vi "swiatla drogowe.vi"() -> ()   [LabVIEW 2025]
uses:
  Semafor1.ctl
  zmienna stanu.ctl
panel:
  in  "OK Button":bool
  out "error out":errorcluster
  in  "number":dbl
  in  "file path (use dialog)":path=path "C:/Users/33sbx/Documents/LABVIEW/światła drogowe/raport.txt"
  out "concatenated string":string
  in  "Zapisz":bool
  out "S4":T1
  out "Obecna sekwencja":T2
  out "S3":T1
  out "S2":T1
  out "S1":T1
  out "Waveform Chart":dbl(graph)
  in  "Reset":bool
  out "Parametr J":dbl
  in  "STOP":bool
  out "OPC22":bool
  out "OPC21":bool
  out "OPZ21":bool
  out "OPZ22":bool
  in  "OPA22":bool
  in  "OPA21":bool
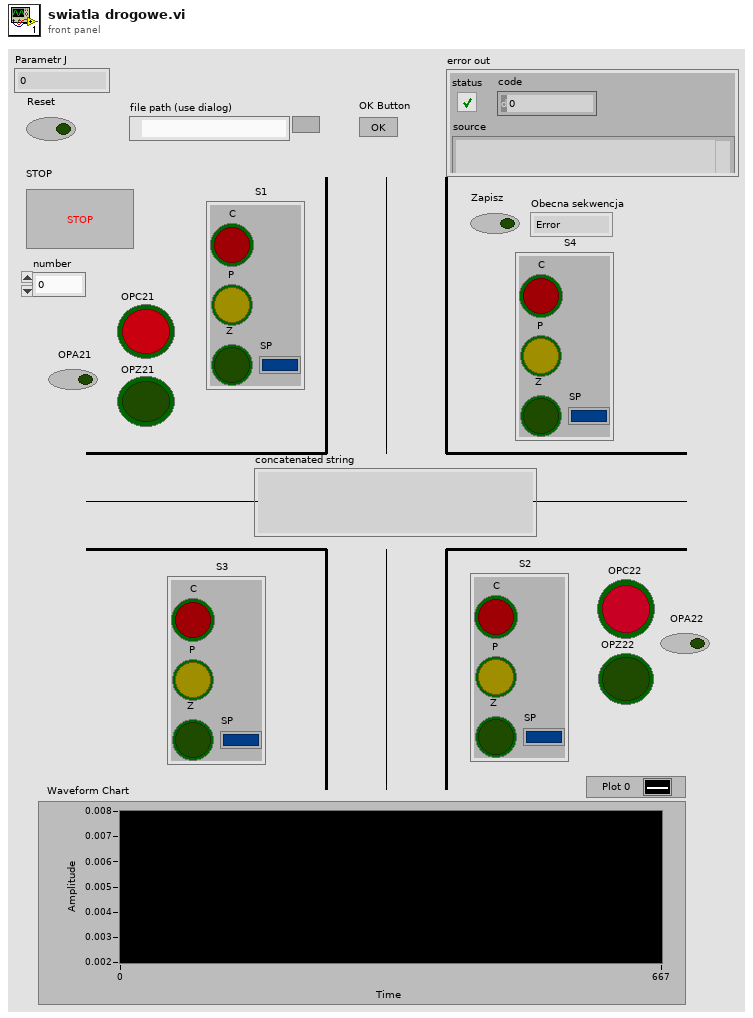
[diagram p1: front panel]
types:
  T1 = typedef "Semafor1.ctl" = cluster{"C":bool, "P":bool, "Z":bool, "SP":bool}
  T2 = typedef "zmienna stanu.ctl" = enum16{"Error", "KGczerwony", "KGpomarañczowy", "KGzielony", "KGpom-czer", "KPpom-czer", "KPzielony", "KPpomarañczowy", "KGczerwony2", "KPpom-czer2", "AwariaON", "AwariaOFF", ""}
  T3 = enum16{"open", "replace", "create", "open or create", "replace or create", "replace or create with confirmation"}
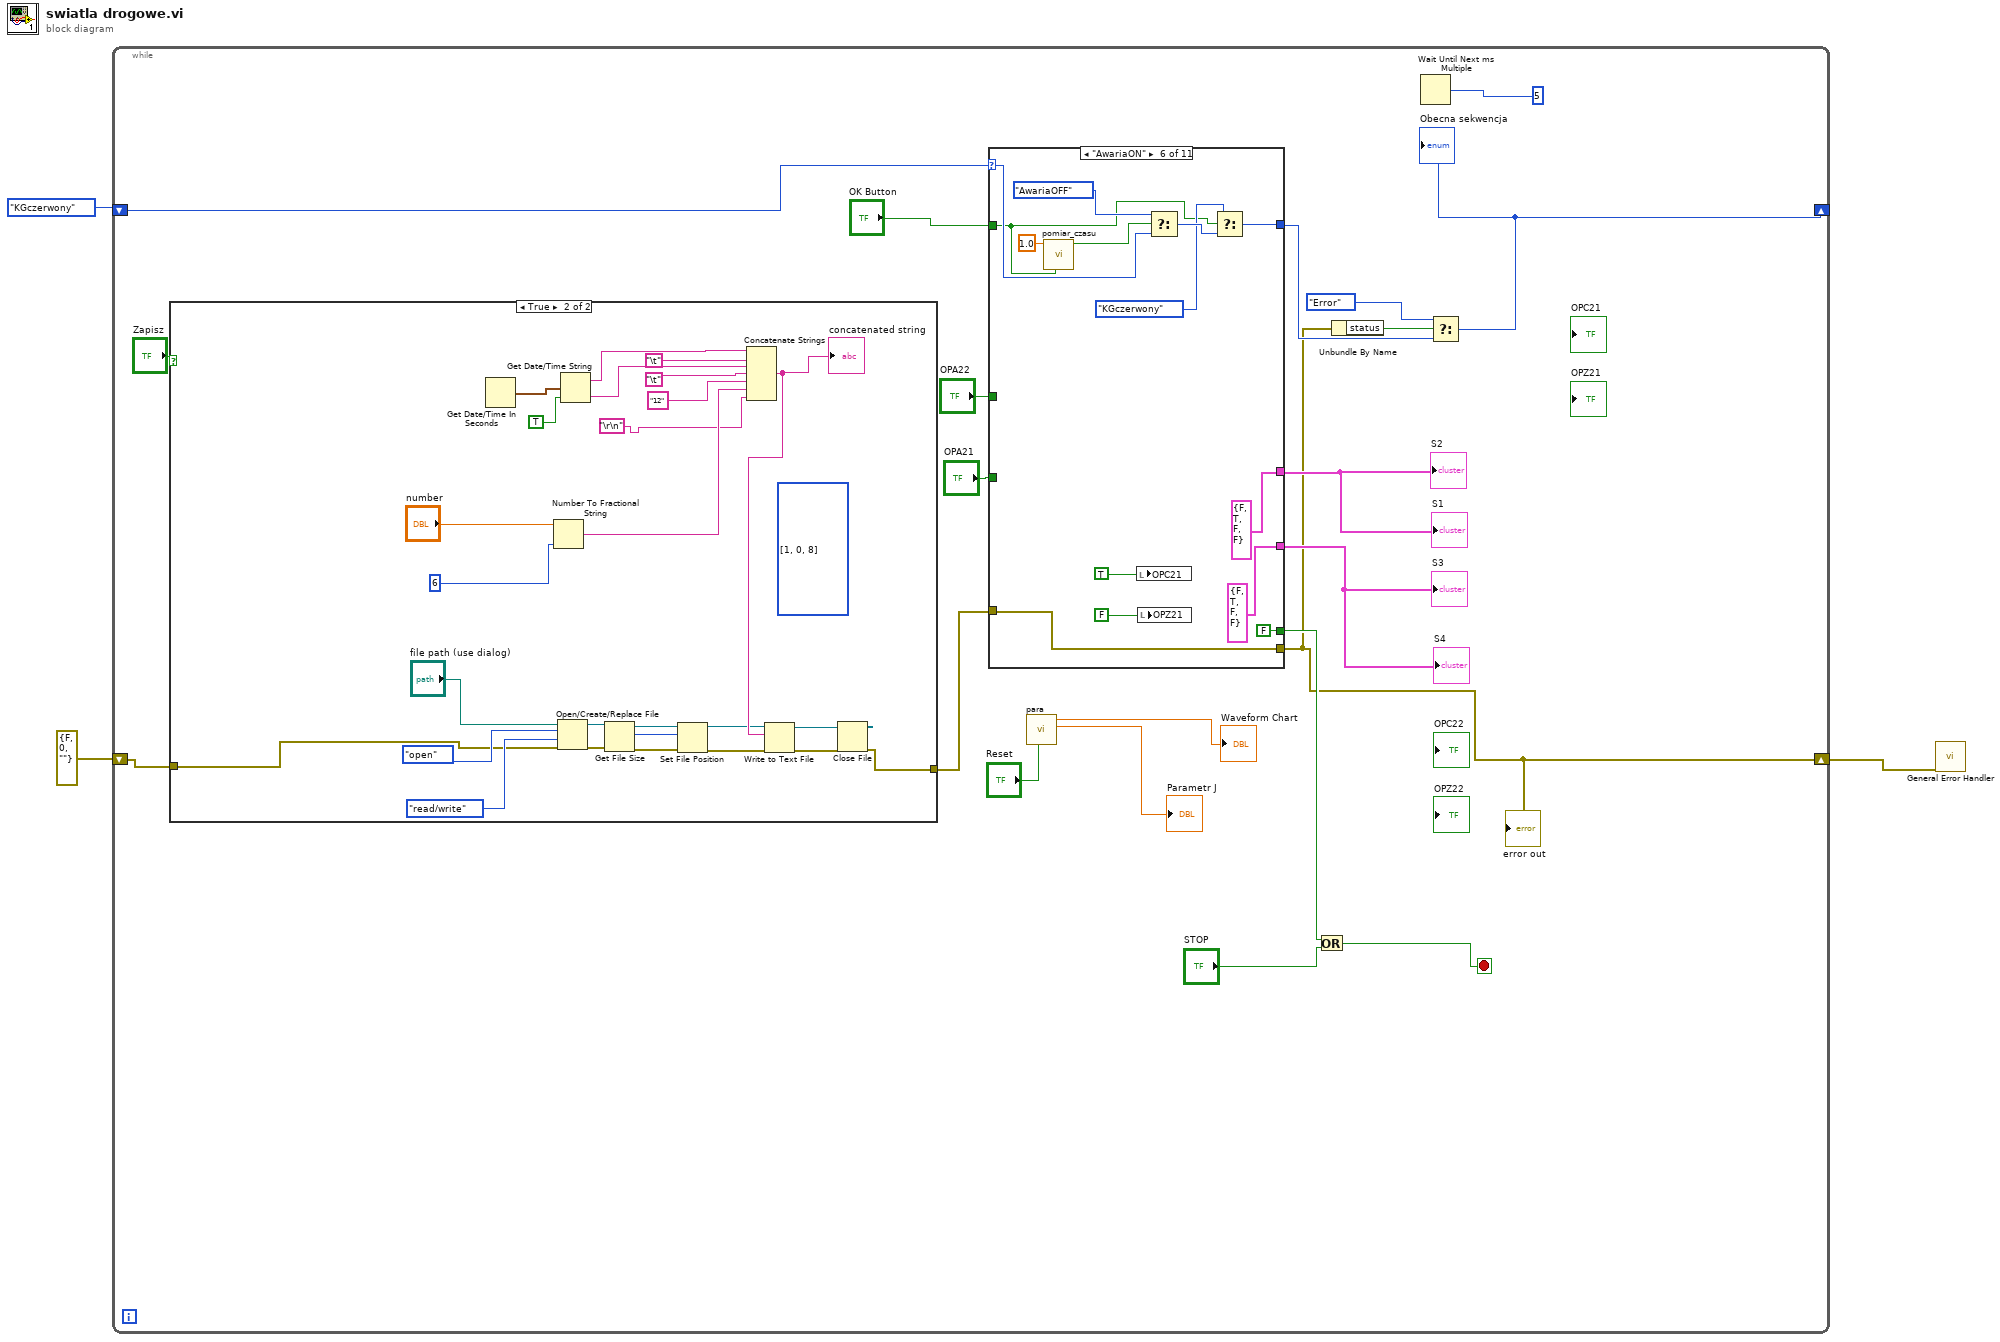
[diagram p0: block diagram]
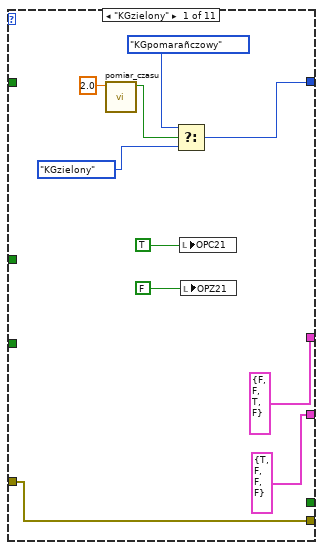
[diagram p3: hidden frame]
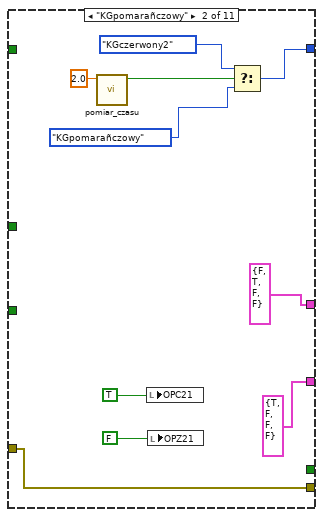
[diagram p4: hidden frame]
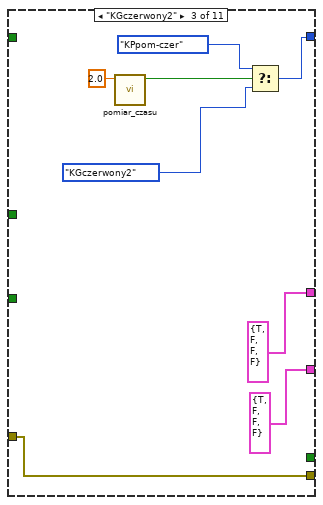
[diagram p5: hidden frame]
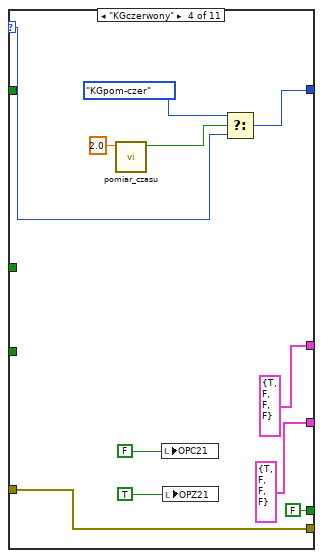
[diagram p6: hidden frame]
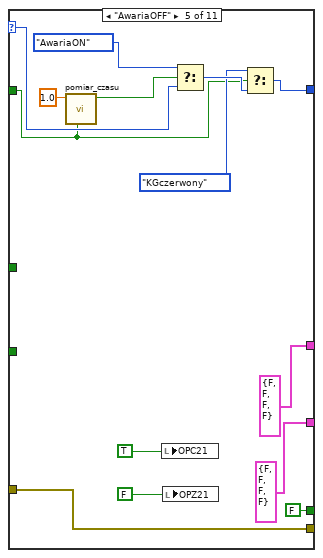
[diagram p7: hidden frame]
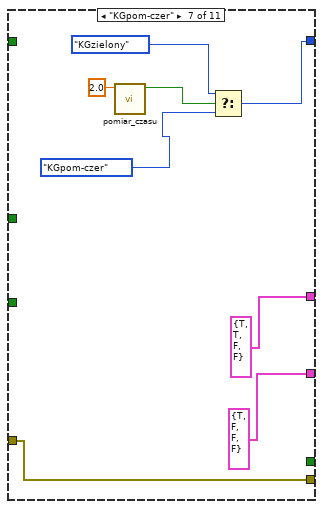
[diagram p8: hidden frame]
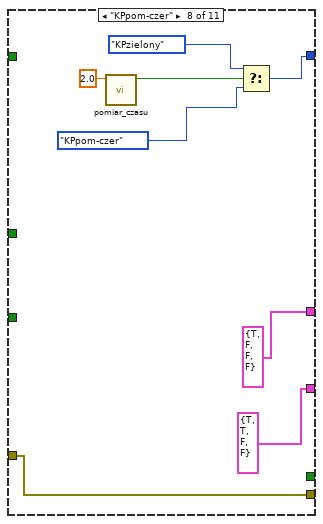
[diagram p9: hidden frame]
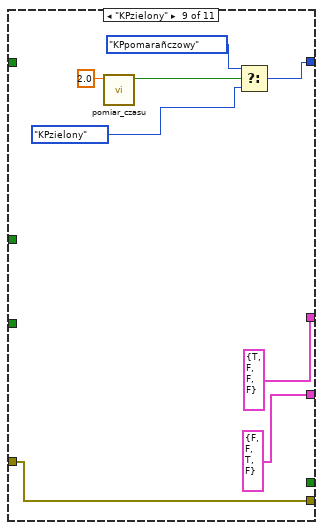
[diagram p10: hidden frame]
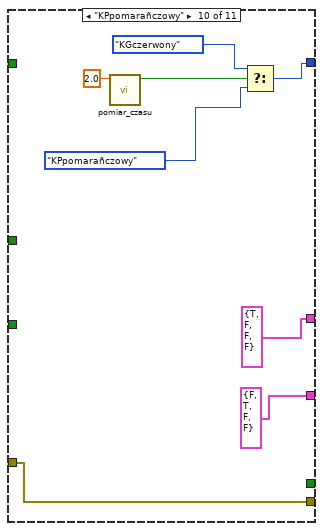
[diagram p11: hidden frame]
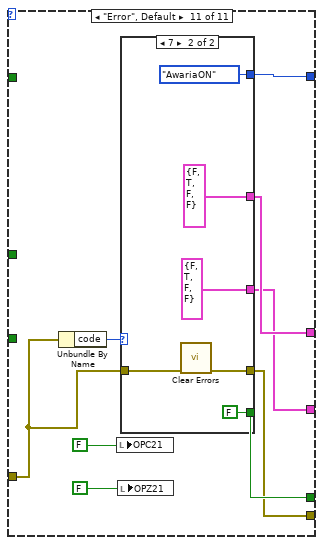
[diagram p12: hidden frame]
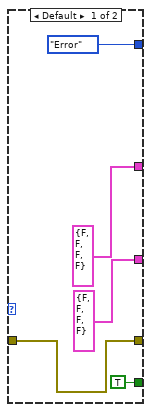
[diagram p13: hidden frame]
diagram:
  n1 = while {
    shift-right: [w10] -> _
    shift-left: zmienna_stanu."KGczerwony" -> [w23]
    shift-right: [w5] -> w1
    shift-left: errorcluster {"status"=FALSE, "code"=0, "source"=""} ("error constant") -> [w13]
    stop <- w7 stop-if-true
    n2 = case shown="True" "Zapisz" {
      tunnel: [w25 w26] -> w14
      tunnel: w13 -> [w25 w31]
      frame False {
      }
      frame True {
        (unwired) u8[] [1, 0, 8]
        n3 = Get Date/Time In Seconds() -> (seconds since 1Jan1904=w51:timestamp)
        n4 = Number To Fractional String(number="number", precision (6)=i16 6) -> (F-format string=w33:string)  [unwired: 2 in]
        n5 = Open/Create/Replace File(file path (use dialog)="file path (use dialog)", error in=w31, operation (0:open)=T3."open", access (0:read/write)=enum16{"read/write", "read-only", "write-only"}."read/write") -> (refnum out=w41:refnum<file>, error out=w30:errorcluster)  [unwired: 2 in, 1 out]
        n6 = Get Date/Time String(seconds (now)=w51, want seconds? (F)=TRUE) -> (date string=w45:string, time string=w48:string)  [unwired: 1 in]
        n7 = Get File Size(file=w41, error in=w30) -> (refnum out=w39:refnum<file>, size (in bytes)=w38:i64, 0:w29:errorcluster)
        n8 = Set File Position(offset (in bytes) (0)=w38, refnum=w39, error in=w29) -> (refnum out=w37:refnum<file>, error out=w28:errorcluster)  [unwired: 1 in]
        n9 = Concatenate Strings(w45, "\t", w48, "\t", "12" ("string"), w33, "\r\n") -> (w42:string)
        "concatenated string" <- w42
        n10 = Write to Text File(file (use dialog)=w37, text=w42, error in=w28) -> (refnum out=w40:refnum<file>, error out=w27:errorcluster)  [unwired: 1 in, 1 out]
        n11 = Close File(refnum=w40, error in=w27) -> (error out=w26:errorcluster)  [unwired: 1 out]
      }
    }
    n12 = case shown="\"AwariaON\"" w23 {
      selector: w23 -> [_ _ _ w84 w99 w113 _ _ _ _ _]
      tunnel: [w59 w68 w76 w85 w94 w106 w122 w129 w137 w147 w151] -> w11
      tunnel: "OPA21" -> [_ _ _ _ _ _ _ _ _ _ _]
      tunnel: [T1 {"C"=FALSE, "P"=FALSE, "Z"=TRUE, "SP"=FALSE} ("S1") T1 {"C"=FALSE, "P"=TRUE, "Z"=FALSE, "SP"=FALSE} ("S1") T1 {"C"=TRUE, "P"=FALSE, "Z"=FALSE, "SP"=FALSE} ("S1") T1 {"C"=TRUE, "P"=FALSE, "Z"=FALSE, "SP"=FALSE} ("S1") T1 {"C"=FALSE, "P"=FALSE, "Z"=FALSE, "SP"=FALSE} ("S1") T1 {"C"=FALSE, "P"=TRUE, "Z"=FALSE, "SP"=FALSE} ("S1") T1 {"C"=TRUE, "P"=TRUE, "Z"=FALSE, "SP"=FALSE} ("S1") T1 {"C"=TRUE, "P"=FALSE, "Z"=FALSE, "SP"=FALSE} ("S1") T1 {"C"=TRUE, "P"=FALSE, "Z"=FALSE, "SP"=FALSE} ("S1") T1 {"C"=TRUE, "P"=FALSE, "Z"=FALSE, "SP"=FALSE} ("S1") w157] -> w18
      tunnel: [T1 {"C"=TRUE, "P"=FALSE, "Z"=FALSE, "SP"=FALSE} ("S4") T1 {"C"=TRUE, "P"=FALSE, "Z"=FALSE, "SP"=FALSE} ("S4") T1 {"C"=TRUE, "P"=FALSE, "Z"=FALSE, "SP"=FALSE} ("S4") T1 {"C"=TRUE, "P"=FALSE, "Z"=FALSE, "SP"=FALSE} ("S4") T1 {"C"=FALSE, "P"=FALSE, "Z"=FALSE, "SP"=FALSE} ("S4") T1 {"C"=FALSE, "P"=TRUE, "Z"=FALSE, "SP"=FALSE} ("S4") T1 {"C"=TRUE, "P"=FALSE, "Z"=FALSE, "SP"=FALSE} ("S4") T1 {"C"=TRUE, "P"=TRUE, "Z"=FALSE, "SP"=FALSE} ("S4") T1 {"C"=FALSE, "P"=FALSE, "Z"=TRUE, "SP"=FALSE} ("S4") T1 {"C"=FALSE, "P"=TRUE, "Z"=FALSE, "SP"=FALSE} ("S4") w156] -> w17
      tunnel: "OPA22" -> [_ _ _ _ _ _ _ _ _ _ _]
      tunnel: [w52 w62 w72 w81 w96 w110 w119 w127 w135 w143 w152] -> w5
      tunnel: w14 -> [w52 w62 w72 w81 w96 w110 w119 w127 w135 w143 w153]
      tunnel: [_ _ _ FALSE ("x") FALSE ("x") FALSE ("x") _ _ _ _ w155] -> w8
      tunnel: "OK Button" -> [_ _ _ _ w91 w105 _ _ _ _ _]
      frame "KGzielony" {
        n13 = call "pomiar_czasu.vi"("czas do odmierzenia"=2.0) -> ("gotowe"=w55:bool)  [unwired: 9 in, 1 out]
        n14 = Select(t=zmienna_stanu."KGpomarañczowy", s=w55, f=zmienna_stanu."KGzielony") -> (s? t:f=w59:T2)
        n15 = local write "OPC21"(TRUE) -> ()
        n16 = local write "OPZ21"(FALSE) -> ()
      }
      frame "KGpomarañczowy" {
        n17 = call "pomiar_czasu.vi"("czas do odmierzenia"=2.0) -> ("gotowe"=w66:bool)  [unwired: 9 in, 1 out]
        n18 = local write "OPC21"(TRUE) -> ()
        n19 = local write "OPZ21"(FALSE) -> ()
        n20 = Select(t=zmienna_stanu."KGczerwony2", s=w66, f=zmienna_stanu."KGpomarañczowy") -> (s? t:f=w68:T2)
      }
      frame "KGczerwony2" {
        n21 = call "pomiar_czasu.vi"("czas do odmierzenia"=2.0) -> ("gotowe"=w78:bool)  [unwired: 9 in, 1 out]
        n22 = Select(t=zmienna_stanu."KPpom-czer", s=w78, f=zmienna_stanu."KGczerwony2") -> (s? t:f=w76:T2)
      }
      frame "KGczerwony" {
        n23 = call "pomiar_czasu.vi"("czas do odmierzenia"=2.0) -> ("gotowe"=w82:bool)  [unwired: 9 in, 1 out]
        n24 = local write "OPC21"(FALSE) -> ()
        n25 = local write "OPZ21"(TRUE) -> ()
        n26 = Select(t=zmienna_stanu."KGpom-czer", s=w82, f=w84) -> (s? t:f=w85:T2)
      }
      frame "AwariaOFF" {
        n27 = call "pomiar_czasu.vi"("Reset"=w91, "czas do odmierzenia"=1.0) -> ("gotowe"=w97:bool)  [unwired: 8 in, 1 out]
        n28 = local write "OPC21"(TRUE) -> ()
        n29 = local write "OPZ21"(FALSE) -> ()
        n30 = Select(t=zmienna_stanu."AwariaON", s=w97, f=w99) -> (s? t:f=w93:T2)
        n31 = Select(t=zmienna_stanu."KGczerwony", s=w91, f=w93) -> (s? t:f=w94:T2)
      }
      frame "AwariaON" {
        n32 = call "pomiar_czasu.vi"("Reset"=w105, "czas do odmierzenia"=1.0) -> ("gotowe"=w111:bool)  [unwired: 8 in, 1 out]
        n33 = local write "OPC21"(TRUE) -> ()
        n34 = local write "OPZ21"(FALSE) -> ()
        n35 = Select(t=zmienna_stanu."AwariaOFF", s=w111, f=w113) -> (s? t:f=w108:T2)
        n36 = Select(t=zmienna_stanu."KGczerwony", s=w105, f=w108) -> (s? t:f=w106:T2)
      }
      frame "KGpom-czer" {
        n37 = call "pomiar_czasu.vi"("czas do odmierzenia"=2.0) -> ("gotowe"=w123:bool)  [unwired: 9 in, 1 out]
        n38 = Select(t=zmienna_stanu."KGzielony", s=w123, f=zmienna_stanu."KGpom-czer") -> (s? t:f=w122:T2)
      }
      frame "KPpom-czer" {
        n39 = call "pomiar_czasu.vi"("czas do odmierzenia"=2.0) -> ("gotowe"=w131:bool)  [unwired: 9 in, 1 out]
        n40 = Select(t=zmienna_stanu."KPzielony", s=w131, f=zmienna_stanu."KPpom-czer") -> (s? t:f=w129:T2)
      }
      frame "KPzielony" {
        n41 = call "pomiar_czasu.vi"("czas do odmierzenia"=2.0) -> ("gotowe"=w139:bool)  [unwired: 9 in, 1 out]
        n42 = Select(t=zmienna_stanu."KPpomarañczowy", s=w139, f=zmienna_stanu."KPzielony") -> (s? t:f=w137:T2)
      }
      frame "KPpomarañczowy" {
        n43 = call "pomiar_czasu.vi"("czas do odmierzenia"=2.0) -> ("gotowe"=w149:bool)  [unwired: 9 in, 1 out]
        n44 = Select(t=zmienna_stanu."KGczerwony", s=w149, f=zmienna_stanu."KPpomarañczowy") -> (s? t:f=w147:T2)
      }
      frame "Error", Default {
        n45 = Unbundle By Name(w153) -> ("code"=w154:i32)
        n46 = local write "OPC21"(FALSE) -> ()
        n47 = local write "OPZ21"(FALSE) -> ()
        n48 = case shown="7" w154 {
          tunnel: [T1 {"C"=FALSE, "P"=FALSE, "Z"=FALSE, "SP"=FALSE} ("S1") T1 {"C"=FALSE, "P"=TRUE, "Z"=FALSE, "SP"=FALSE} ("S1")] -> w157
          tunnel: [T1 {"C"=FALSE, "P"=FALSE, "Z"=FALSE, "SP"=FALSE} ("S4") T1 {"C"=FALSE, "P"=TRUE, "Z"=FALSE, "SP"=FALSE} ("S4")] -> w156
          tunnel: [TRUE ("x") FALSE ("x")] -> w155
          tunnel: [w161 w165] -> w152
          tunnel: w153 -> [w161 w166]
          tunnel: [zmienna_stanu."Error" zmienna_stanu."AwariaON"] -> w151
          frame Default {
          }
          frame 7 {
            n49 = call <vilib>:"Clear Errors.vi"("error in (no error)"=w166) -> ("error out"=w165:errorcluster)  [unwired: 5 in, 1 out]
          }
        }
      }
    }
    "S1" <- w18
    "S2" <- w18
    "S3" <- w17
    "S4" <- w17
    "error out" <- w5
    n50 = call "para.vi"("Reset"="Reset") -> ("Parametr J"=→"Parametr J":dbl, "czas cyklu"=→"Waveform Chart":dbl)  [unwired: 9 in]
    n51 = Or(x=w8, y="STOP") -> (x .or. y?=w7:bool)
    n52 = Unbundle By Name(w5) -> ("status"=w6:bool)
    n53 = Wait Until Next ms Multiple(millisecond multiple=5) -> ()  [unwired: 1 out]
    n54 = Select(t=zmienna_stanu."Error", s=w6, f=w11) -> (s? t:f=w10:T2)
    "Obecna sekwencja" <- w10
  }
  n55 = call <vilib>:"General Error Handler.vi"("error in (no error)"=w1) -> ()  [unwired: 10 in, 5 out]
